vi "GetText.vi"(8 "error in":errorcluster, 11 "J1939 editor node in":refnum<class "J1939 editor node.lvclass">) -> (0 "error out":errorcluster, 1 "additional text":string, 2 "text":string, 3 "J1939 editor node out":refnum<class "J1939 editor node.lvclass">, 4 "glyph":string)   [LabVIEW 2013, in "J1939 editor node.lvclass"]
doc: "Use this VI to display the name of the module in the tree and to specify the desired glyph in the configuration editor."
uses:
  J1939 editor node.lvclass
  <vilib>/NI/DCAF/Tag Editor Core/Configuration Editor/Classes/Module editor node/Read display name.vi
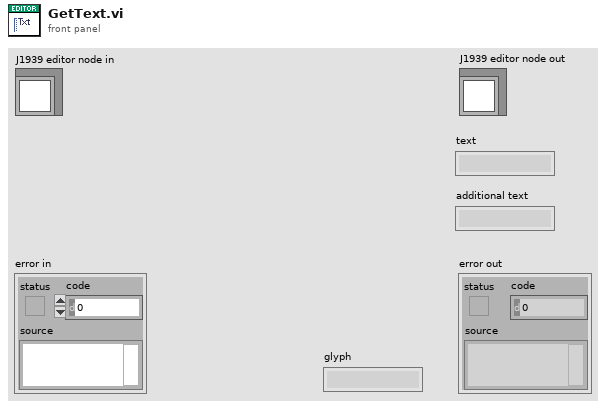
[diagram p1: front panel]
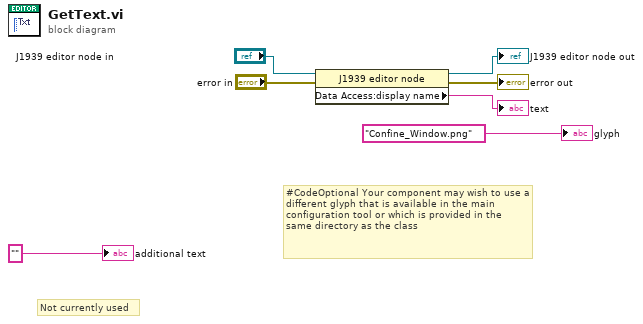
[diagram p0: block diagram]
diagram:
  # "Not currently used"
  # "#CodeOptional Your component may wish to use a different glyph that is available in the main configuration tool or which is provided in the same directory as the class"
  n1 = property class="J1939 editor node"(reference="J1939 editor node in", error in="error in") -> (reference out=→"J1939 editor node out":refnum<class "J1939 editor node.lvclass">, error out=→"error out":errorcluster, "Data Access:display name"=→"text":string)
  "additional text" <- "" ("additional text")
  "glyph" <- "Confine_Window.png" ("glyph")
